vi "Catapult open.vi"() -> (0 "error out":errorcluster, 3 "Catapult devrevs":T3)   [LabVIEW 2013]
uses:
  <vilib>/Rock Robotics/SystemInterfaces/Typedef/FPGA_TypedefDigitalModule.ctl
  <vilib>/Rock Robotics/SystemInterfaces/DIO/FPGA_DIOPWMChannel.ctl
  <vilib>/Rock Robotics/SystemInterfaces/DIO/FPGA_DIOChannel.ctl
  catapult type def.ctl
  <vilib>/Rock Robotics/WPI/MotorControl/WPI_MotorControlDeviceRef.ctl
  <vilib>/Rock Robotics/WPI/PWM/WPI_PWMDeadband.ctl
  <vilib>/Rock Robotics/WPI/CAN/Jaguar/SubVIs/WPI_CANJaguar_ControlMode.ctl
  <vilib>/Rock Robotics/WPI/PWM/WPI_PWMTransform_ConPane.ctl
  <vilib>/Rock Robotics/WPI/Solenoid/WPI_SolenoidDevRef.ctl
  <vilib>/Rock Robotics/SystemInterfaces/Typedef/FPGA_TypedefSolenoidModule.ctl
  <vilib>/Rock Robotics/WPI/Solenoid/WPI_SolenoidChannel.ctl
  <vilib>/Rock Robotics/WPI/DigitalInput/WPI_DigitalInputDevRef.ctl
  <vilib>/Rock Robotics/WPI/Solenoid/WPI_SolenoidOpenDouble.vi
  <vilib>/Rock Robotics/WPI/MotorControl/WPI_MotorControlOpen Talon.vi
panel:
  in  "second limit":T1=enum."DIO 5"
  in  "Reverse Wench Channel":T2=enum."Solenoid 4"
  in  "Forward Wench Channel":T2=enum."Solenoid 3"
  in  "first limit":T1=enum."DIO 4"
  in  "PWM Channel":T6=enum."PWM 4"
  in  "Digital Module (Module 1)":T5
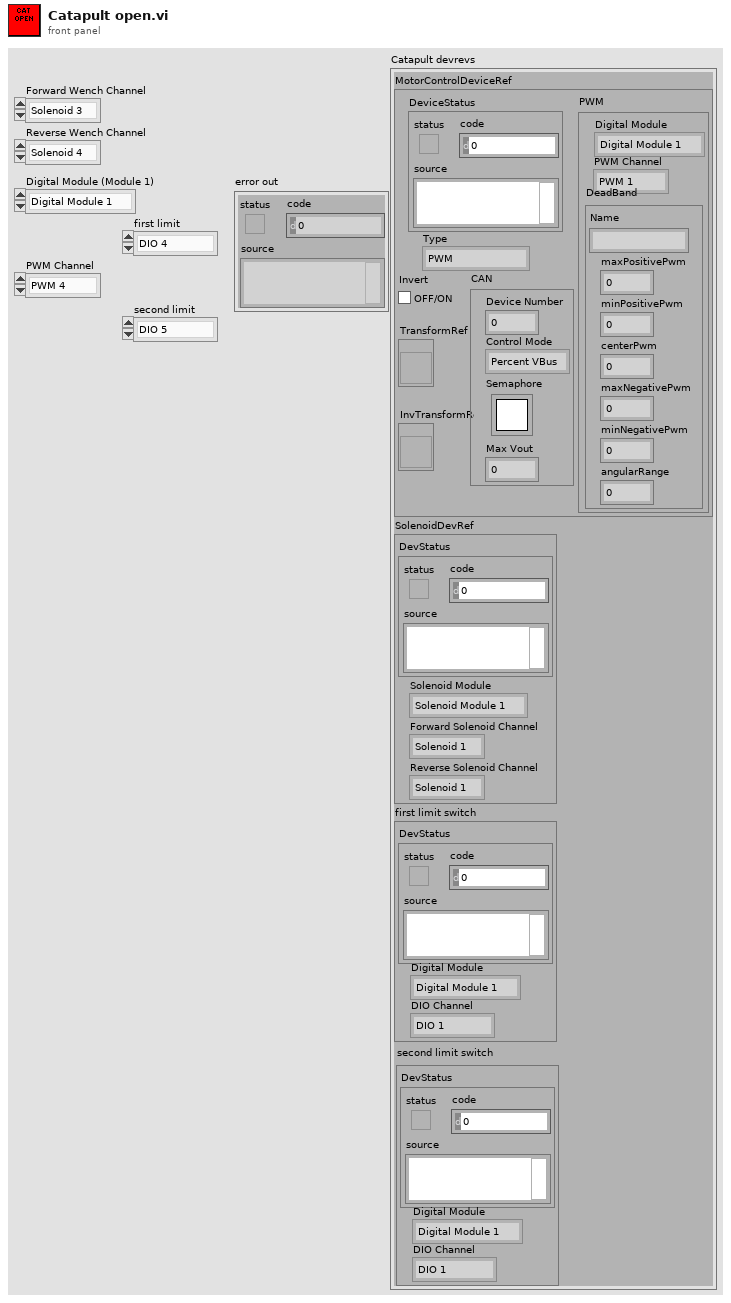
[diagram p1: front panel]
types:
  T1 = typedef "FPGA_DIOChannel.ctl" = enum8{"DIO 1", "DIO 2", "DIO 3", "DIO 4", "DIO 5", "DIO 6", "DIO 7", "DIO 8", "DIO 9", "DIO 10", "DIO 11", "DIO 12", "DIO 13", "DIO 14", "Invalid"}
  T2 = typedef "WPI_SolenoidChannel.ctl" = enum8{"Solenoid 1", "Solenoid 2", "Solenoid 3", "Solenoid 4", "Solenoid 5", "Solenoid 6", "Solenoid 7", "Solenoid 8", "Invalid"}
  T3 = typedef "catapult type def.ctl" = cluster{"MotorControlDeviceRef":T4, "SolenoidDevRef":T11, "first limit switch":T13, "second limit switch":T13}
  T4 = typedef "WPI_MotorControlDeviceRef.ctl" = cluster{"DeviceStatus":errorcluster, "Type":enum16{"PWM", "CAN"}, "PWM":cluster{"Digital Module":T5, "PWM Channel":T6, "DeadBand":T7}, "CAN":cluster{"Device Number":u8, "Control Mode":T8, "Semaphore":T9, "Max Vout":dbl}, "Invert":bool, "TransformRef":T10, "InvTransformRef":T10}
  T5 = typedef "FPGA_TypedefDigitalModule.ctl" = enum16{"Digital Module 1", "Digital Module 2"}
  T6 = typedef "FPGA_DIOPWMChannel.ctl" = enum8{"PWM 1", "PWM 2", "PWM 3", "PWM 4", "PWM 5", "PWM 6", "PWM 7", "PWM 8", "PWM 9", "PWM 10", "Invalid"}
  T7 = typedef "WPI_PWMDeadband.ctl" = cluster{"Name":string, "maxPositivePwm":i32, "minPositivePwm":i32, "centerPwm":i32, "maxNegativePwm":i32, "minNegativePwm":i32, "angularRange":u16}
  T8 = typedef "WPI_CANJaguar_ControlMode.ctl" = enum8{"Percent VBus", "Current", "Speed", "Position", "Voltage"}
  T9 = typedef "Semaphore RefNum" = refnum<k1>
  T10 = typedef "WPI_PWMTransform_ConPane.ctl" = refnum<vi>
  T11 = typedef "WPI_SolenoidDevRef.ctl" = cluster{"DevStatus":errorcluster, "Solenoid Module":T12, "Forward Solenoid Channel":T2, "Reverse Solenoid Channel":T2}
  T12 = typedef "FPGA_TypedefSolenoidModule.ctl" = enum16{"Solenoid Module 1", "Solenoid Module 2"}
  T13 = typedef "WPI_DigitalInputDevRef.ctl" = cluster{"DevStatus":errorcluster, "DIO Channel":T1, "Digital Module":T5}
  T14 = cluster{"MotorControlDeviceRef":T4, "SolenoidDevRef":T11, "DigitalInputDevRef":T13, "DigitalInputDevRef":T13}
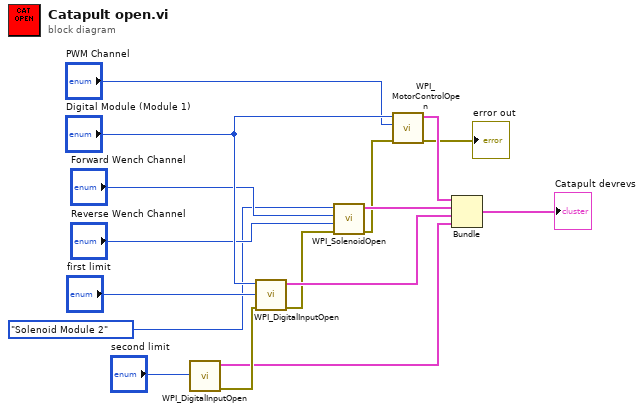
[diagram p0: block diagram]
diagram:
  n1 = call <vilib>:"WPI_DigitalInputOpen.vi"("DIO Channel"="second limit") -> ("error out"=w4:errorcluster, "DigitalInputDevRef"=w3:T13)  [unwired: 9 in]
  n2 = call <vilib>:"WPI_DigitalInputOpen.vi"("error in (no error)"=w4, "DIO Channel"="first limit", "Digital Module (Module 1)"="Digital Module (Module 1)") -> ("error out"=w10:errorcluster, "DigitalInputDevRef"=w14:T13)  [unwired: 7 in]
  n3 = call-poly <vilib>:"WPI_SolenoidOpen.vi"("error in (no error)"=w10, "Reverse Solenoid Channel"="Reverse Wench Channel", "Forward Solenoid Channel"="Forward Wench Channel", "Solenoid Module (Module 1)"=FPGA_TypedefSolenoidModule."Solenoid Module 2") -> ("error out"=w9:errorcluster, "SolenoidDevRef"=w15:T11)  [unwired: 6 in]
  n4 = call-poly <vilib>:"WPI_MotorControlOpen.vi"("error in (no error)"=w9, "PWM Channel"="PWM Channel", "Digital Module (Module 1)"="Digital Module (Module 1)") -> ("error out"=→"error out":errorcluster, "MotorControlDeviceRef"=w16:T4)  [unwired: 7 in]
  n5 = Bundle("MotorControlDeviceRef"=w16, "SolenoidDevRef"=w15, "DigitalInputDevRef"=w14, "DigitalInputDevRef"=w3) -> (→"Catapult devrevs":T14)  [unwired: 1 in]
